vi "read log.vi"() -> ()   [LabVIEW 2020]
uses:
  <vilib>/Utility/sysdir.llb/System Directory Type.ctl
  <vilib>/addons/_JKI Toolkits/State Machine/_JKI_lib_State_Machine.llb/Select State(s)_err__jki_lib_state_machine.vi
  <vilib>/JDP Science/JSONtext/JSONtext.lvlib
panel:
  in  "refresh":bool
  in  "Log Files":i32(listbox)
  out "message":string
  in  "timestamp":i32(listbox)
  in  "Exit":bool
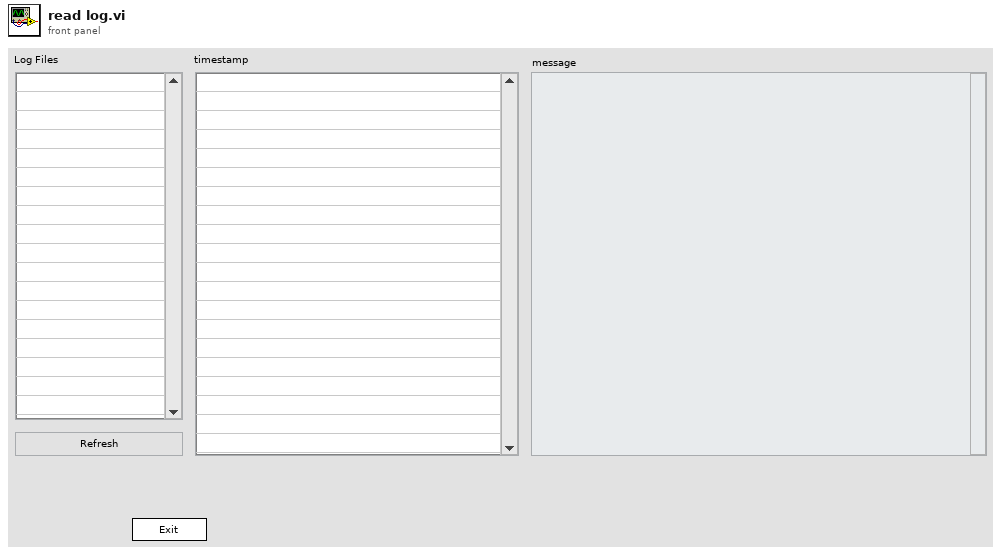
[diagram p1: front panel]
types:
  T1 = enum32{"Invalid", "Standard", "Closed", "Hidden", "Minimized", "Maximized"}
  T2 = enum32{"invalid app kind", "Development System", "Run Time System", "Student Edition", "Embedded LabVIEW", "Evaluation", "Custom"}
  T3 = cluster{"Core":cluster{"Current VI Reference":refnum<vi>, "Close Panel on Exit?":bool}, "log file":path, "elements":string[], "Log Directory":path}
  T4 = typedef "System Directory Type.ctl" = i32
  T5 = cluster{"Current VI Reference":refnum<vi>, "Close Panel on Exit?":bool}
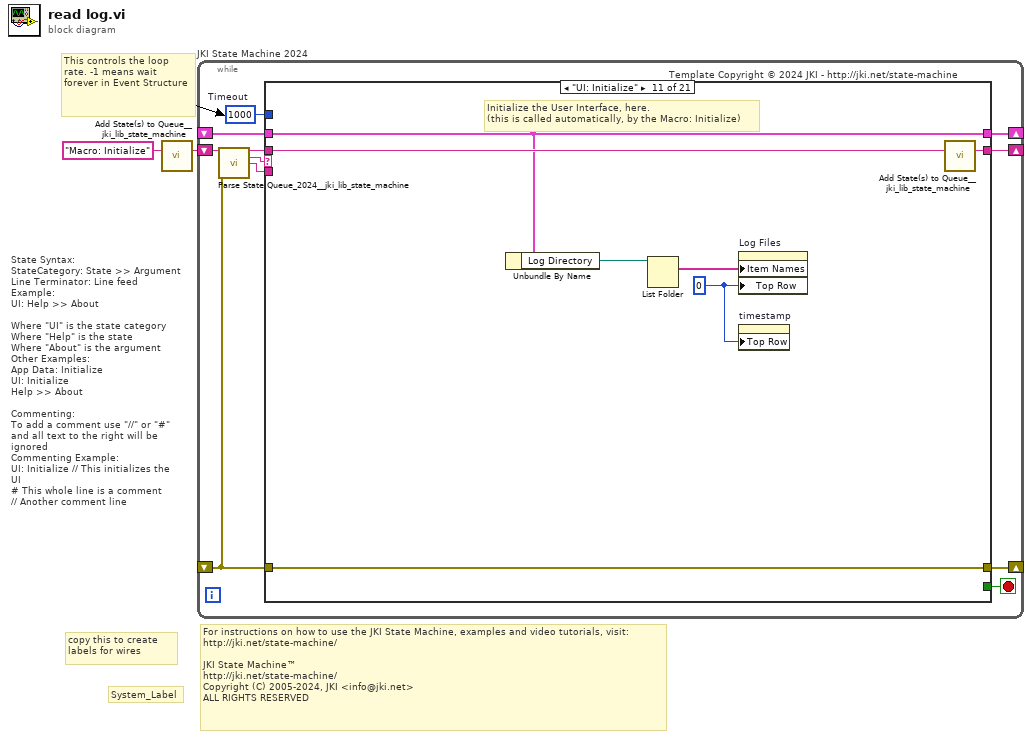
[diagram p0: block diagram]
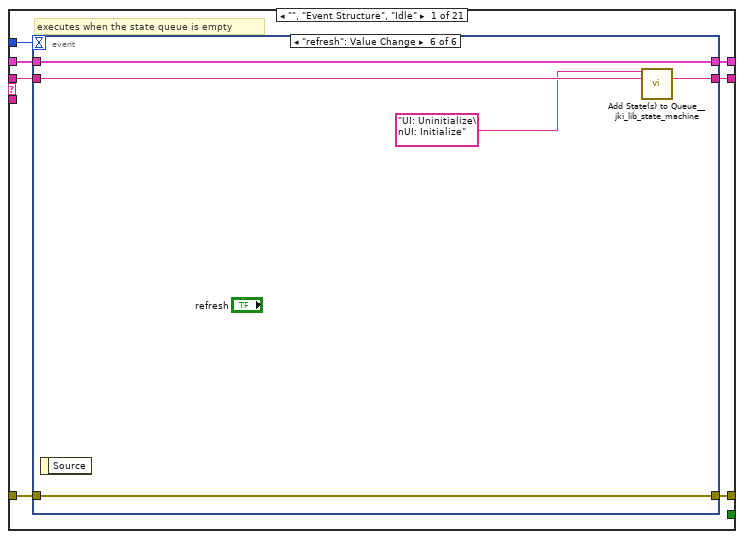
[diagram p2: hidden frame]
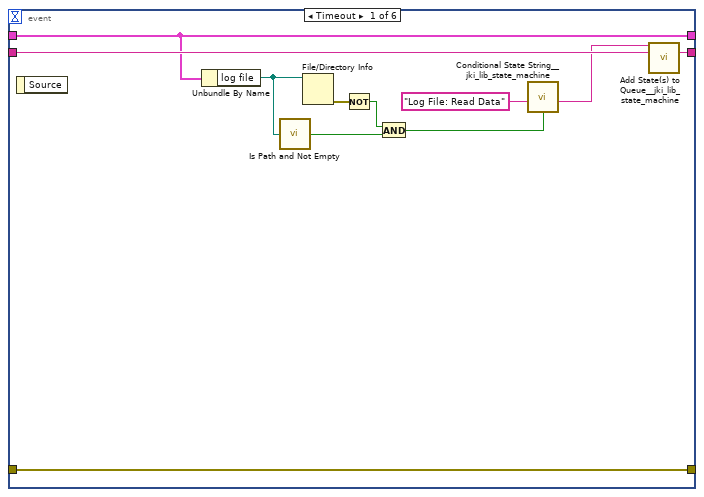
[diagram p3: hidden frame]
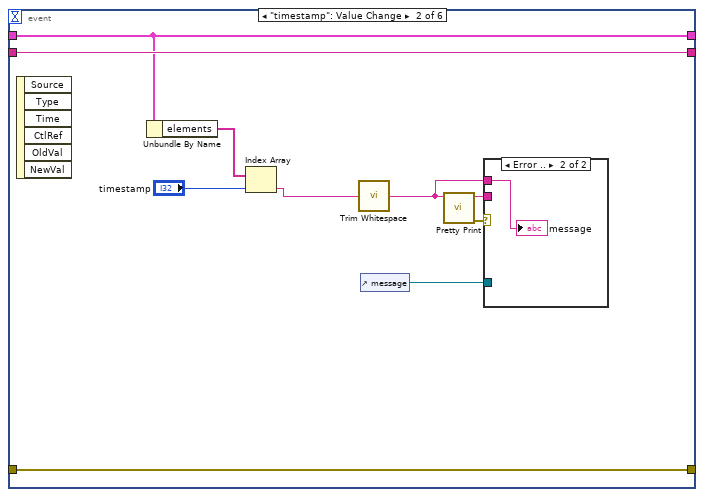
[diagram p4: hidden frame]
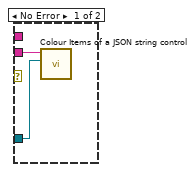
[diagram p5: hidden frame]
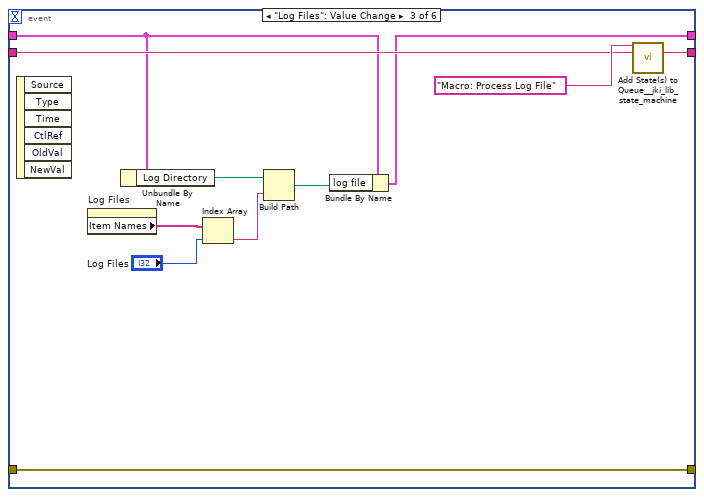
[diagram p6: hidden frame]
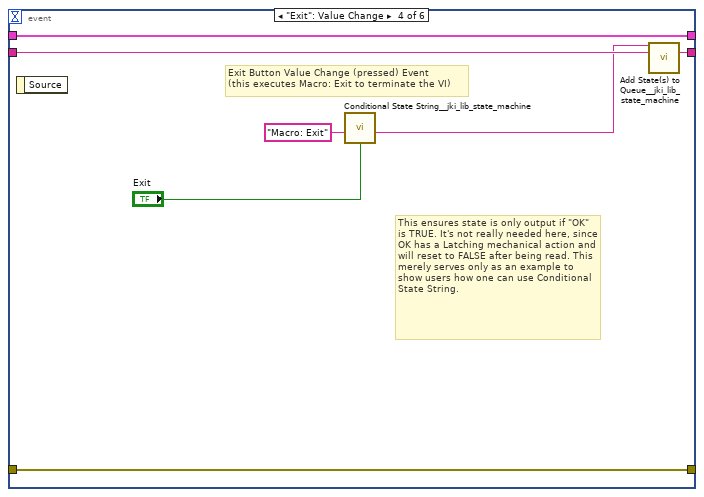
[diagram p7: hidden frame]
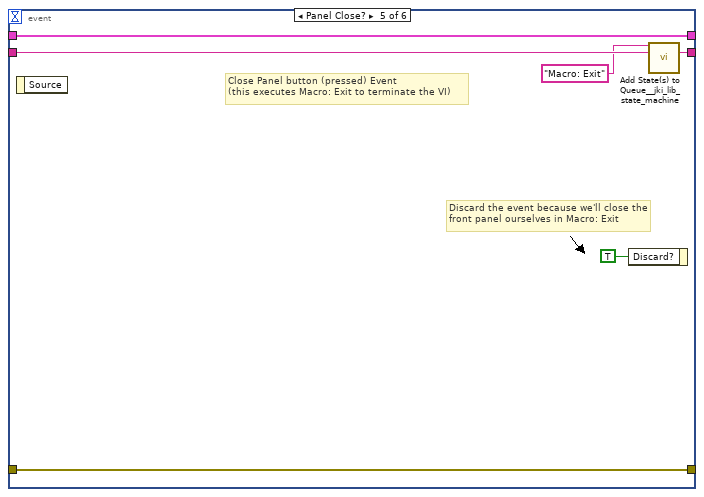
[diagram p8: hidden frame]
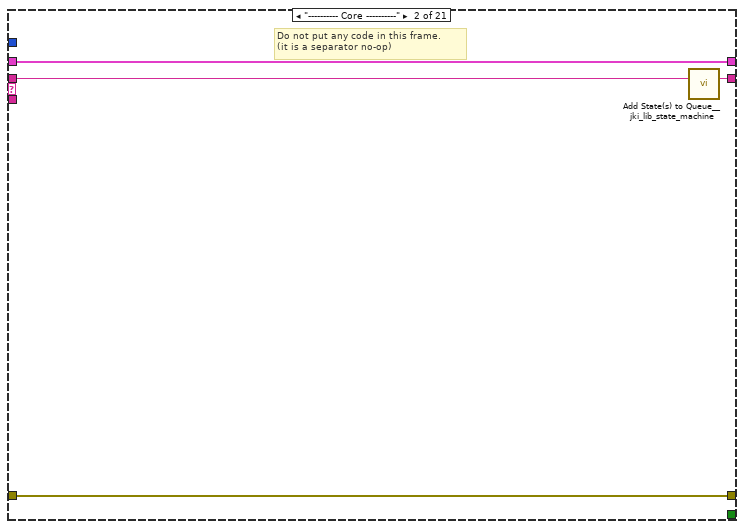
[diagram p9: hidden frame]
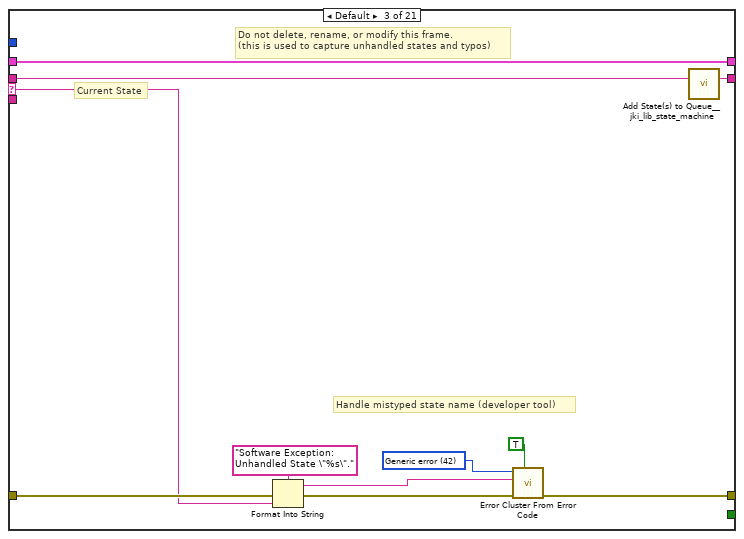
[diagram p10: hidden frame]
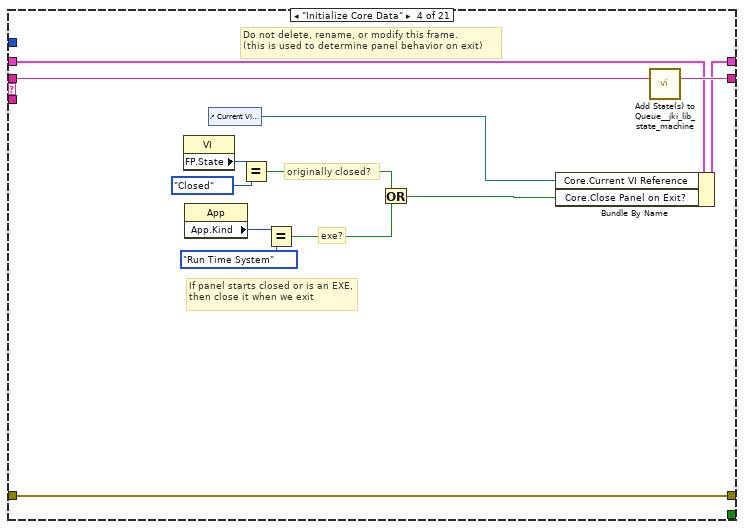
[diagram p11: hidden frame]
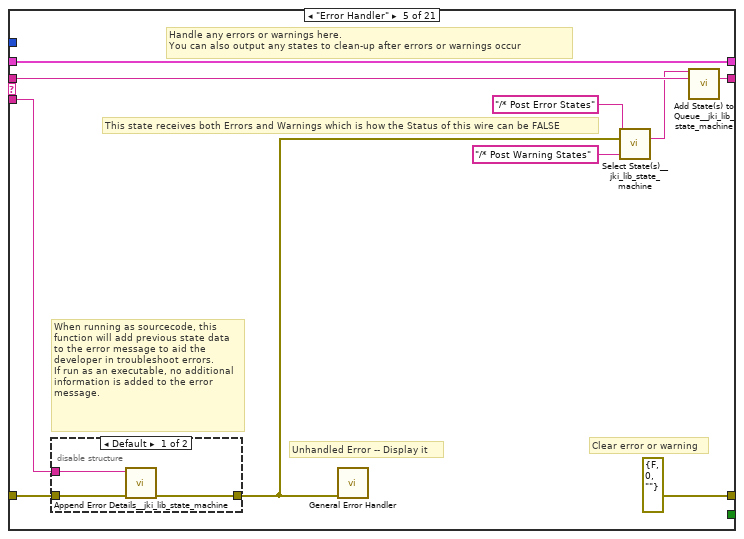
[diagram p12: hidden frame]
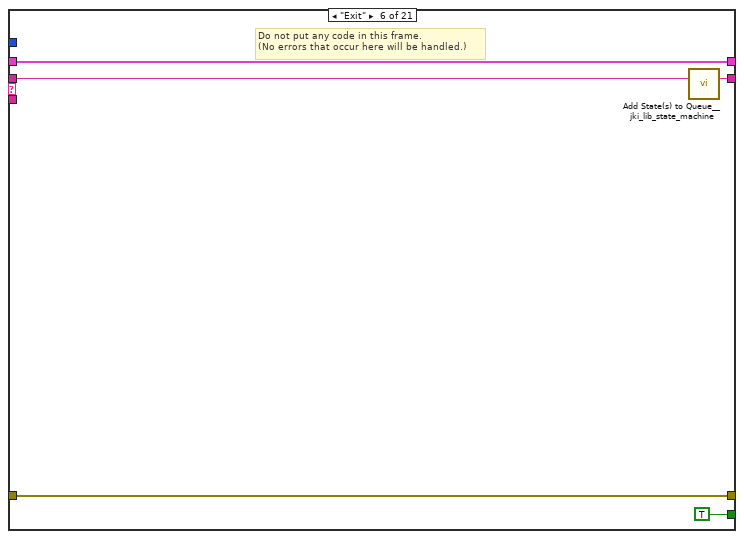
[diagram p14: hidden frame]
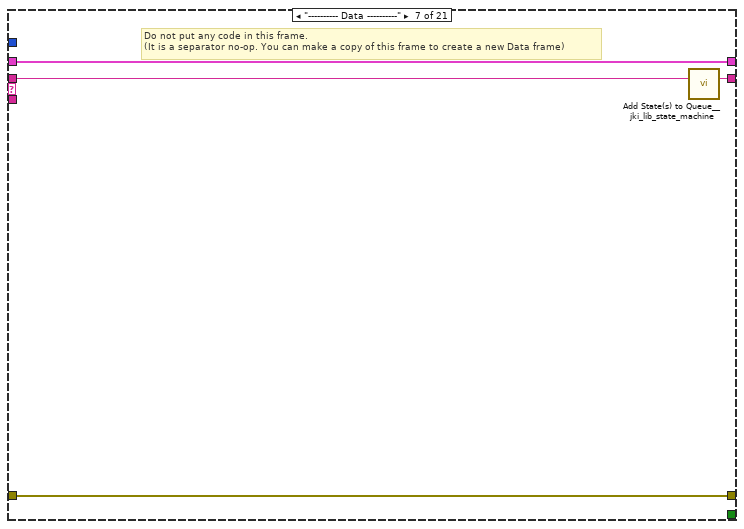
[diagram p15: hidden frame]
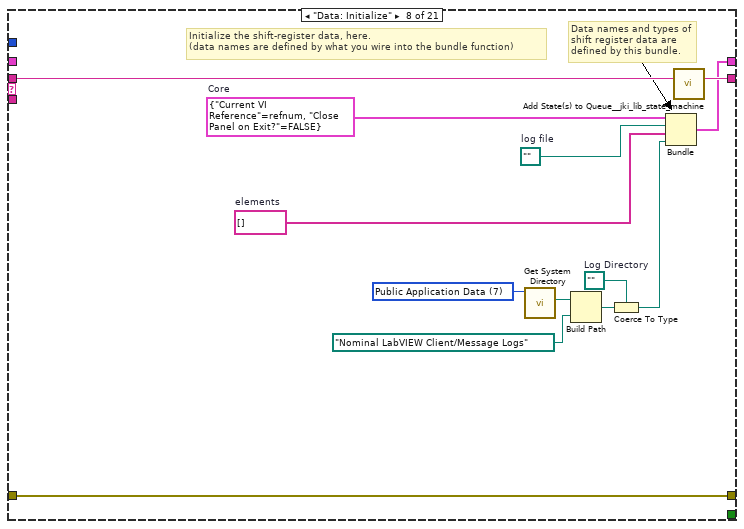
[diagram p16: hidden frame]
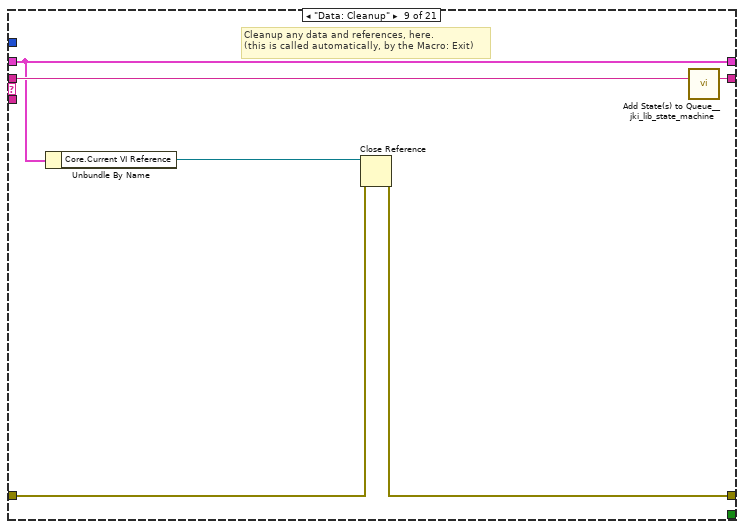
[diagram p17: hidden frame]
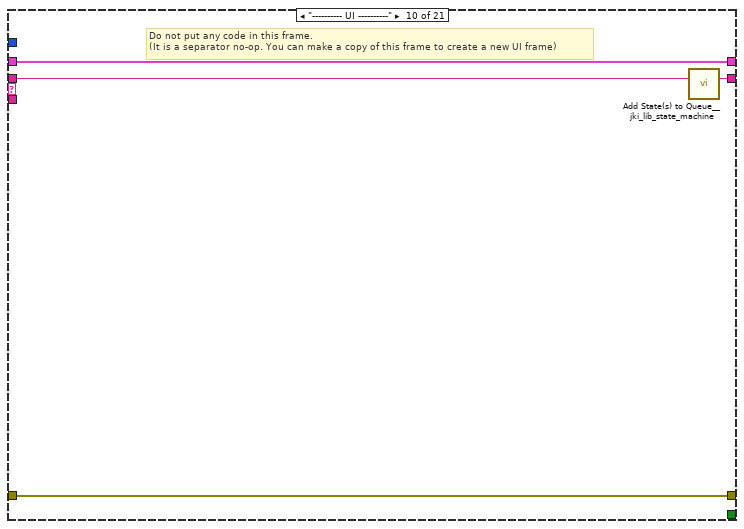
[diagram p18: hidden frame]
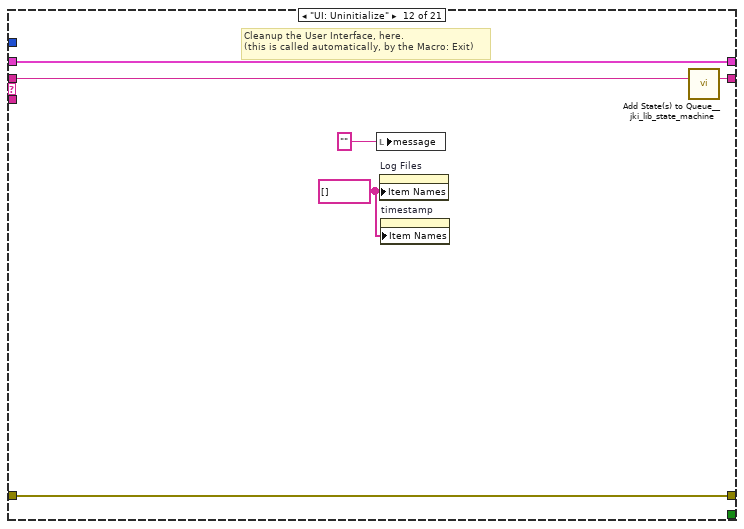
[diagram p19: hidden frame]
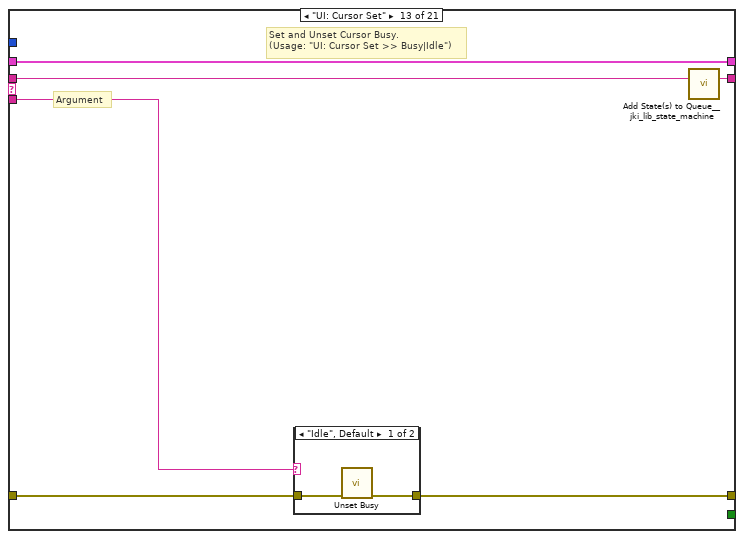
[diagram p20: hidden frame]
diagram:
  # "For instructions on how to use the JKI State Machine, examples and video tutorials, visit:\nhttp://jki.net/state-machine/\n\nJKI State Machine™\nhttp://jki.net/state-machine/\nCopyright (C) 2005-2024, JKI <info@jki.net>\nALL RIGHTS RESERVED"
  # "State Syntax:\nStateCategory: State >> Argument\nLine Terminator: Line feed\nExample:\nUI: Help >> About\n\nWhere \"UI\" is the state category\nWhere \"Help\" is the state\nWhere \"About\" is the argument\nOther Examples:\nApp Data: Initialize\nUI: Initialize\nHelp >> About\n\nCommenting:\nTo add a comment use \"//\" or \"#\" and all text to the right will be ignored\nCommenting Example:\nUI: Initialize // This initializes the UI\n# This whole line is a comment\n// Another comment line"
  # "copy this to create labels for wires"
  # "This controls the loop rate. -1 means wait forever in Event Structure"
  # "System_Label"
  n1 = call <vilib>:"Add State(s) to Queue__jki_lib_state_machine.vi"("State(s) in (\"\")"="Macro: Initialize") -> ("States Out"=w2:string)  [unwired: 14 in]
  n2 = while "JKI State Machine 2024" {
    shift-right: [w6] -> _
    shift-left: _ -> [w5]
    shift-right: [w9] -> _
    shift-left: _ -> [w3]
    shift-right: [w8] -> _
    shift-left: w2 -> [w10]
    stop <- w7 stop-if-true
    w4 = 1000  # Timeout
    # "Template Copyright © 2024 JKI - http://jki.net/state-machine"
    n3 = call <vilib>:"Parse State Queue_2024__jki_lib_state_machine.vi"("State Queue"=w10, "Error In (no error)"=w3) -> ("Remaining States"=w12:string, "Current State"=w13:string, "Arguments"=w11:string)  [unwired: 11 in]
    n4 = case shown="\"UI: Initialize\"" w13 {
      selector: w13 -> [_ _ w78 _ _ _ _ _ _ _ _ _ _ _ _ _ _ _ _ _ _]
      tunnel: w12 -> [w20 w77 w82 w101 w111 w120 w124 w137 w143 w147 w154 w155 w166 w177 w246 w251 w260 w265 w269 w285 w302]
      tunnel: w11 -> [_ _ _ _ w106 _ _ _ _ _ _ _ w161 w171 _ _ _ _ _ _ _]
      tunnel: w5 -> [w18 w74 w80 w94 w108 w118 w121 _ w138 w144 w150 w159 w164 w173 w243 w248 w258 w263 w266 w272 w299]
      tunnel: [w17 w75 w84 w98 errorcluster {"status"=FALSE, "code"=0, "source"=""} ("error out") w117 w122 w134 w139 w145 w152 w158 w162 w174 w244 w249 w255 w262 w267 w278 w300] -> w9
      tunnel: w3 -> [w14 w75 w83 w98 w107 w117 w122 w134 w140 w145 w152 w158 w163 w175 w244 w249 w255 w262 w267 w277 w300]
      tunnel: [w19 w76 w81 w100 w110 w119 w123 w136 w142 w146 w153 w160 w165 w176 w245 w250 w259 w264 w268 w284 w301] -> w8
      tunnel: [_ _ _ _ _ TRUE _ _ _ _ _ _ _ _ _ _ _ _ _ _ _] -> w7
      tunnel: [w16 w74 w80 w99 w108 w118 w121 w135 w138 w144 w150 w159 w164 w173 w243 w248 w258 w263 w266 w271 w299] -> w6
      tunnel: w4 -> [w15 _ _ _ _ _ _ _ _ _ _ _ _ _ _ _ _ _ _ _ _]
      frame "", "Event Structure", "Idle" {
        # "executes when the state queue is empty"
        n5 = event shown="[5] \"refresh\": Value Change" {
          selector: _ -> [_ _ _ _ _ _]
          dyn-events: _ -> [_ _ _ _ _ _]
          timeout: w15 -> [_ _ _ _ _ _]
          tunnel: w20 -> [w31 w41 w53 w62 w68 w71]
          tunnel: [w30 w41 w52 w61 w67 w72] -> w19
          tunnel: w18 -> [w28 w40 w47 w59 w65 w73]
          tunnel: [w29 w33 w55 w60 w66 w70] -> w17
          tunnel: w14 -> [w29 w33 w55 w60 w66 w70]
          tunnel: [w28 w40 w45 w59 w65 w73] -> w16
          event Timeout {
            n6 = event-data() -> ()  [unwired: 1 in, 1 out]
            n7 = Unbundle By Name(w28) -> ("log file"=w26:path)
            n8 = call <vilib>:"Is Path and Not Empty.vi"("path"=w26) -> ("Is Path and Not Empty?"=w25:bool)  [unwired: 4 in]
            n9 = File/Directory Info(path=w26) -> (error out=w27:errorcluster)  [unwired: 1 in, 6 out]
            n10 = Not(x=w27) -> (.not. x?=w24:bool)
            n11 = And(x=w24, y=w25) -> (x .and. y?=w22:bool)
            n12 = call <vilib>:"Conditional State String__jki_lib_state_machine.vi"("Do State(s)?"=w22, "State"="Log File: Read Data") -> ("State Out"=w23:string)  [unwired: 7 in]
            n13 = call <vilib>:"Add State(s) to Queue__jki_lib_state_machine.vi"("State(s) in Front (\"\")"=w23, "State(s) in (\"\")"=w31) -> ("States Out"=w30:string)  [unwired: 13 in]
          }
          event "timestamp": Value Change {
            n14 = event-data() -> ()  [unwired: 1 in, 6 out]
            n15 = Unbundle By Name(w40) -> ("elements"=w39:string[])
            n16 = Index Array(array=w39, index="timestamp") -> (element=w32:string)
            n17 = call <vilib>:"Trim Whitespace.vi"("string"=w32) -> ("trimmed string"=w34:string)  [unwired: 1 in]
            n18 = control-ref of="message"() -> (w37:refnum<vi>)
            n19 = call <vilib>:"Pretty Print.vi"("JSON"=w34) -> ("error out"=w35:errorcluster, "<JSON>"=w36:string)  [unwired: 8 in, 1 out]
            n20 = case shown="Error .." w35 {
              tunnel: w37 -> [w43 _]
              tunnel: w36 -> [w42 _]
              tunnel: w34 -> [_ w44]
              frame No Error {
                n21 = call <vilib>:"Colour Items of a JSON string control.vi"("String Control"=w43, "JSON"=w42) -> ()  [unwired: 9 in, 1 out]
              }
              frame Error {
                "message" <- w44
              }
            }
          }
          event "Log Files": Value Change {
            n22 = event-data() -> ()  [unwired: 1 in, 6 out]
            n23 = property on="Log Files" class="LstBox (strict)"() -> ("Item Names"=w50:string[])  [unwired: 2 in, 2 out]
            n24 = Unbundle By Name(w47) -> ("Log Directory"=w51:path)
            n25 = Index Array(array=w50, index="Log Files") -> (element=w48:string)
            n26 = Build Path(base path=w51, name or relative path=w48) -> (appended path=w46:path)
            n27 = Bundle By Name(cluster=w47, "log file"=w46) -> (w45:T3)
            n28 = call <vilib>:"Add State(s) to Queue__jki_lib_state_machine.vi"("State(s) in Front (\"\")"="Macro: Process Log File" ("string"), "State(s) in (\"\")"=w53) -> ("States Out"=w52:string)  [unwired: 13 in]
          }
          event "Exit": Value Change {
            # "This ensures state is only output if \"OK\" is TRUE. It's not really needed here, since OK has a Latching mechanical action and will reset to FALSE after being read. This merely serves only as an example to show users how one can use Conditional State String."
            # "Exit Button Value Change (pressed) Event\n(this executes Macro: Exit to terminate the VI)"
            n29 = event-data() -> ()  [unwired: 1 in, 1 out]
            n30 = call <vilib>:"Conditional State String__jki_lib_state_machine.vi"("Do State(s)?"="Exit", "State"="Macro: Exit") -> ("State Out"=w56:string)  [unwired: 7 in]
            n31 = call <vilib>:"Add State(s) to Queue__jki_lib_state_machine.vi"("State(s) in Front (\"\")"=w56, "State(s) in (\"\")"=w62) -> ("States Out"=w61:string)  [unwired: 13 in]
          }
          event Panel Close? {
            # "Discard the event because we'll close the front panel ourselves in Macro: Exit"
            # "Close Panel button (pressed) Event\n(this executes Macro: Exit to terminate the VI)"
            n32 = event-data() -> ()  [unwired: 1 in, 1 out]
            n33 = event-data("Discard?"=TRUE) -> ()  [unwired: 1 in, 1 out]
            n34 = call <vilib>:"Add State(s) to Queue__jki_lib_state_machine.vi"("State(s) in Front (\"\")"="Macro: Exit", "State(s) in (\"\")"=w68) -> ("States Out"=w67:string)  [unwired: 13 in]
          }
          event "refresh": Value Change {
            n35 = event-data() -> ()  [unwired: 1 in, 1 out]
            n36 = call <vilib>:"Add State(s) to Queue__jki_lib_state_machine.vi"("State(s) in Front (\"\")"="UI: Uninitialize\nUI: Initialize" ("State(s) in Front (\"\")"), "State(s) in (\"\")"=w71) -> ("States Out"=w72:string)  [unwired: 13 in]
          }
        }
      }
      frame "---------- Core ----------" {
        # "Do not put any code in this frame.\n(it is a separator no-op)"
        n37 = call <vilib>:"Add State(s) to Queue__jki_lib_state_machine.vi"("State(s) in (\"\")"=w77) -> ("States Out"=w76:string)  [unwired: 14 in]
      }
      frame Default {
        w87 = 42 items=["No error", "Argument error", "Memory is full", "Out of zone", "End of file", "File already open", "Generic file I/O error", "File not found", "File permission error", "Disk is full", "Duplicate path", "Too many files open", "System feature not enabled", "Resource file not found", "Cannot add resource", "Resource not found", "Image not found", "Image memory error", "Pen does not exist", "Config type invalid", "Config token not found", "Config parse error", "Config memory error", "Bad external code format", "Bad external code offset", "External code not present", "Null window", "Destroy window error", "Null menu", "Print aborted", "Bad print record", "Print driver error", "Windows error during printing", "Memory error during printing", "Print dialog error", "Generic print error", "Invalid device refnum", "Device not found", "Device parameter error", "Device unit error", "Cannot open device", "Device call aborted", "Generic error", "Cancelled by user", "Object ID too low", "Object ID too high", "Object not in heap", "Unknown heap", "Unknown object (invalid DefProc)", "Unknown object (DefProc not in table)", "Message out of range", "Invalid (null) method", "Unknown message", "Manager call not supported", "Bad address", "Network operation in progress", "Network operation timed out", "Connection is busy", "Network attribute not supported", "Network error", "Address in use", "System out of memory", "Connection aborted", "Connection refused", "Not connected", "Already connected", "Connection closed", "Initialization error (interapplication manager)", "Bad occurrence", "Wait on unbound occurrence handler", "Occurrence queue overflow", "Datalog type conflict", "Unused", "Unrecognized type (interapplication manager)", "Memory corrupt", "Failed to make temporary DLL", "Old CIN version", "Drag socket not found", "Failed to load drop-object", "Failed to register OLE object", "Failed to release OLE object", "Format specifier type mismatch", "Unknown format specifier", "Too few format specifiers", "Too many format specifiers", "Scan failed", "Newer CIN version", "Error converting to variant", "Runtime menu error", "Password tampered", "Variant attribute not found", "Incompatible variant data type", "Event data is not available", "Event Store is not present", "Occurrence is not found", "Event Queue is not created", "Event info is not available", "Refnum passed is NULL", "Error retrieving Class GUID", "Error retrieving CoClass GUID", "Error retrieving TypeLib GUID.", "Bad built application magic bytes.", "Specific driver is different from the specific driver associated with the Logical Name.", "There is no session opened to the class driver.", "Max Error", "MAX - Error with config objects", "MAX - Error loading configuration", "MAX - Group not supported"]
        # "Current State"
        # "Do not delete, rename, or modify this frame.\n(this is used to capture unhandled states and typos)"
        # "Handle mistyped state name (developer tool)"
        n38 = Format Into String(format string="Software Exception: Unhandled State \"%s\"." ("message"), error in=w83, w78) -> (resulting string=w86:string, error out=w85:errorcluster)  [unwired: 1 in]
        n39 = call <vilib>:"Error Cluster From Error Code.vi"("show call chain? (False)"=TRUE, "error in (no error)"=w85, "error message (\"\")"=w86, "error code (0)"=w87) -> ("error out"=w84:errorcluster)  [unwired: 5 in]
        n40 = call <vilib>:"Add State(s) to Queue__jki_lib_state_machine.vi"("State(s) in (\"\")"=w82) -> ("States Out"=w81:string)  [unwired: 14 in]
      }
      frame "Initialize Core Data" {
        # "Do not delete, rename, or modify this frame.\n(this is used to determine panel behavior on exit)"
        # "originally closed?"
        # "exe?"
        # "If panel starts closed or is an EXE, then close it when we exit"
        n41 = property class="VI"() -> ("FP.State"=w91:T1)  [unwired: 2 in, 2 out]
        n42 = property class="App"() -> ("App.Kind"=w97:T2)  [unwired: 2 in, 2 out]
        n43 = control-ref of="Current VI Reference"() -> (w92:refnum<vi>)
        n44 = Equal?(x=w91, y=T1."Closed" ("Front Panel Window:State")) -> (x = y?=w89:bool)
        n45 = Equal?(x=w97, y=T2."Run Time System" ("Application:Kind")) -> (x = y?=w95:bool)
        n46 = Or(x=w89, y=w95) -> (x .or. y?=w93:bool)
        n47 = Bundle By Name(cluster=w94, "Core.Current VI Reference"=w92, "Core.Close Panel on Exit?"=w93) -> (w99:T3)
        n48 = call <vilib>:"Add State(s) to Queue__jki_lib_state_machine.vi"("State(s) in (\"\")"=w101) -> ("States Out"=w100:string)  [unwired: 14 in]
      }
      frame "Error Handler" {
        # "When running as sourcecode, this function will add previous state data to the error message to aid the developer in troubleshoot errors.\nIf run as an executable, no additional information is added to the error message."
        # "This state receives both Errors and Warnings which is how the Status of this wire can be FALSE"
        # "Unhandled Error -- Display it"
        # "Handle any errors or warnings here.\nYou can also output any states to clean-up after errors or warnings occur"
        # "Clear error or warning"
        n49 = disable-structure shown="Default" {
          disable-tunnel: w107 -> [w114 w115]
          disable-tunnel: w106 -> [w113 _]
          disable-tunnel: [w112 w115] -> w105
          frame condition #0 (active) {
            n50 = call <vilib>:"Append Error Details__jki_lib_state_machine.vi"("error in (no error)"=w114, "Previous State and Argument(s)"=w113) -> ("error out"=w112:errorcluster)  [unwired: 9 in]
          }
          frame condition #1 {
          }
        }
        n51 = call <vilib>:"General Error Handler.vi"("error in (no error)"=w105) -> ()  [unwired: 10 in, 5 out]
        n52 = call-poly <vilib>:"Select State(s)__jki_lib_state_machine.vi"("State(s) if True (\"\")"="/* Post Error States", "Select"=w105, "State(s) if False (\"\")"="/* Post Warning States") -> ("States Out"=w103:string)  [unwired: 12 in]
        n53 = call <vilib>:"Add State(s) to Queue__jki_lib_state_machine.vi"("State(s) in Front (\"\")"=w103, "State(s) in (\"\")"=w111) -> ("States Out"=w110:string)  [unwired: 13 in]
      }
      frame "Exit" {
        # "Do not put any code in this frame.\n(No errors that occur here will be handled.)"
        n54 = call <vilib>:"Add State(s) to Queue__jki_lib_state_machine.vi"("State(s) in (\"\")"=w120) -> ("States Out"=w119:string)  [unwired: 14 in]
      }
      frame "---------- Data ----------" {
        # "Do not put any code in this frame.\n(It is a separator no-op. You can make a copy of this frame to create a new Data frame)"
        n55 = call <vilib>:"Add State(s) to Queue__jki_lib_state_machine.vi"("State(s) in (\"\")"=w124) -> ("States Out"=w123:string)  [unwired: 14 in]
      }
      frame "Data: Initialize" {
        w125 = path ""  # Log Directory
        w130 = T4 7 items=["User Home"=0, "User Desktop"=1, "User Documents"=2, "User Application Data"=3, "User Preferences"=4, "User Temporary"=5, "Public Documents"=6, "Public Application Data"=7, "Public Preferences"=8, "Public Cache"=13, "System Core Libraries"=9, "System Installed Libraries"=10, "Application Files"=11, "Boot Volume Root"=12] ("system directory type")
        w131 = string[] []  # elements
        w132 = path ""  # log file
        w133 = T5 {"Current VI Reference"=refnum, "Close Panel on Exit?"=FALSE}  # Core
        # "Data names and types of shift register data are defined by this bundle."
        # "Initialize the shift-register data, here.\n(data names are defined by what you wire into the bundle function)"
        n56 = call <vilib>:"Get System Directory.vi"("system directory type"=w130) -> ("system directory"=w129:path)  [unwired: 10 in]
        n57 = Build Path(base path=w129, name or relative path=path "Nominal LabVIEW Client/Message Logs") -> (appended path=w127:path)
        n58 = Coerce To Type(0:w127, 1:w125) -> (2:w126:path)
        n59 = Bundle("Core"=w133, "log file"=w132, "elements"=w131, "Log Directory"=w126) -> (w135:T3)  [unwired: 1 in]
        n60 = call <vilib>:"Add State(s) to Queue__jki_lib_state_machine.vi"("State(s) in (\"\")"=w137) -> ("States Out"=w136:string)  [unwired: 14 in]
      }
      frame "Data: Cleanup" {
        # "Cleanup any data and references, here.\n(this is called automatically, by the Macro: Exit)"
        n61 = Unbundle By Name(w138) -> ("Core.Current VI Reference"=w141:refnum<vi>)
        n62 = Close Reference(reference=w141, error in (no error)=w140) -> (error out=w139:errorcluster)
        n63 = call <vilib>:"Add State(s) to Queue__jki_lib_state_machine.vi"("State(s) in (\"\")"=w143) -> ("States Out"=w142:string)  [unwired: 14 in]
      }
      frame "---------- UI ----------" {
        # "Do not put any code in this frame.\n(It is a separator no-op. You can make a copy of this frame to create a new UI frame)"
        n64 = call <vilib>:"Add State(s) to Queue__jki_lib_state_machine.vi"("State(s) in (\"\")"=w147) -> ("States Out"=w146:string)  [unwired: 14 in]
      }
      frame "UI: Initialize" {
        w148 = 0 ("Top Row")
        # "Initialize the User Interface, here.\n(this is called automatically, by the Macro: Initialize)"
        n65 = Unbundle By Name(w150) -> ("Log Directory"=w149:path)
        n66 = List Folder(path=w149) -> (filenames=w151:string[])  [unwired: 3 in, 3 out]
        n67 = property on="Log Files" class="LstBox (strict)"("Item Names"=w151, "Top Row"=w148) -> ()  [unwired: 2 in, 2 out]
        n68 = property on="timestamp" class="LstBox (strict)"("Top Row"=w148) -> ()  [unwired: 2 in, 2 out]
        n69 = call <vilib>:"Add State(s) to Queue__jki_lib_state_machine.vi"("State(s) in (\"\")"=w154) -> ("States Out"=w153:string)  [unwired: 14 in]
      }
      frame "UI: Uninitialize" {
        w157 = string[] [] ("Item Names")
        # "Cleanup the User Interface, here.\n(this is called automatically, by the Macro: Exit)"
        n70 = local write "message"("") -> ()
        n71 = property on="Log Files" class="LstBox (strict)"("Item Names"=w157) -> ()  [unwired: 2 in, 2 out]
        n72 = property on="timestamp" class="LstBox (strict)"("Item Names"=w157) -> ()  [unwired: 2 in, 2 out]
        n73 = call <vilib>:"Add State(s) to Queue__jki_lib_state_machine.vi"("State(s) in (\"\")"=w155) -> ("States Out"=w160:string)  [unwired: 14 in]
      }
      frame "UI: Cursor Set" {
        # "Argument"
        # "Set and Unset Cursor Busy.\n(Usage: \"UI: Cursor Set >> Busy|Idle\")"
        n74 = case shown="\"Idle\", Default" w161 {
          tunnel: w163 -> [w168 w170]
          tunnel: [w167 w169] -> w162
          frame "Idle", Default {
            n75 = call <vilib>:"Unset Busy.vi"("error in (no error)"=w168) -> ("error out"=w167:errorcluster)  [unwired: 10 in]
          }
          frame "Busy" {
            n76 = call <vilib>:"Set Busy.vi"("error in (no error)"=w170) -> ("error out"=w169:errorcluster)  [unwired: 9 in, 1 out]
          }
        }
        n77 = call <vilib>:"Add State(s) to Queue__jki_lib_state_machine.vi"("State(s) in (\"\")"=w166) -> ("States Out"=w165:string)  [unwired: 14 in]
      }
      frame "UI: Front Panel State" {
        # "Argument"
        # "Set Front Panel Open or Closed\n(Usage: \"UI: Front Panel State >> Open|Close\")"
        n78 = Unbundle By Name(w173) -> ("Core.Current VI Reference"=w172:refnum<vi>)
        n79 = case shown="\"Minimize\", \"Minimized\"" w171 {
          tunnel: w175 -> [w183 w198 w209 w222 w235]
          tunnel: [w185 w199 w211 w224 w237] -> w174
          tunnel: w172 -> [w184 w196 w210 w223 w236]
          frame "Open", "Standard", Default {
            w178 = T1."Standard" ("State")
            n80 = property class="VI"(reference=w184, error in=w183) -> (reference out=w181:refnum<vi>, error out=w182:errorcluster, "FP.State"=w180:T1)
            n81 = Not Equal?(x=w180, y=w178) -> (x != y?=w179:bool)
            n82 = case shown="True" w179 {
              tunnel: [w189 w191] -> w185
              tunnel: w182 -> [w188 w191]
              tunnel: w181 -> [w187 _]
              tunnel: w178 -> [w186 _]
              frame True {
                n83 = invoke class="VI" method="FP.Open"(reference=w187, error in=w188, "Activate"=TRUE, "State"=w186) -> (error out=w189:errorcluster)  [unwired: 1 in, 4 out]
              }
              frame False {
              }
            }
          }
          frame "Close", "Closed" {
            n84 = property class="VI"(reference=w196, error in=w198) -> (reference out=w195:refnum<vi>, error out=w197:errorcluster, "FP.State"=w193:T1)
            n85 = Not Equal?(x=w193, y=T1."Closed" ("Front Panel Window:State")) -> (x != y?=w192:bool)
            n86 = case shown="True" w192 {
              tunnel: [w200 w203] -> w199
              tunnel: w197 -> [w200 w202]
              tunnel: w195 -> [_ w201]
              frame False {
              }
              frame True {
                n87 = invoke class="VI" method="FP.Close"(reference=w201, error in=w202) -> (error out=w203:errorcluster)  [unwired: 1 in, 2 out]
              }
            }
          }
          frame "Hidden", "Hide" {
            w204 = T1."Hidden" ("State")
            n88 = property class="VI"(reference=w210, error in=w209) -> (reference out=w207:refnum<vi>, error out=w208:errorcluster, "FP.State"=w206:T1)
            n89 = Not Equal?(x=w206, y=w204) -> (x != y?=w205:bool)
            n90 = case shown="True" w205 {
              tunnel: [w215 w216] -> w211
              tunnel: w208 -> [w214 w216]
              tunnel: w207 -> [w213 _]
              tunnel: w204 -> [w212 _]
              frame True {
                n91 = invoke class="VI" method="FP.Open"(reference=w213, error in=w214, "State"=w212) -> (error out=w215:errorcluster)  [unwired: 2 in, 4 out]
              }
              frame False {
              }
            }
          }
          frame "Minimize", "Minimized" {
            w217 = T1."Minimized" ("State")
            n92 = property class="VI"(reference=w223, error in=w222) -> (reference out=w220:refnum<vi>, error out=w221:errorcluster, "FP.State"=w219:T1)
            n93 = Not Equal?(x=w219, y=w217) -> (x != y?=w218:bool)
            n94 = case shown="True" w218 {
              tunnel: [w228 w229] -> w224
              tunnel: w221 -> [w227 w229]
              tunnel: w220 -> [w226 _]
              tunnel: w217 -> [w225 _]
              frame True {
                n95 = invoke class="VI" method="FP.Open"(reference=w226, error in=w227, "State"=w225) -> (error out=w228:errorcluster)  [unwired: 2 in, 4 out]
              }
              frame False {
              }
            }
          }
          frame "Maximize", "Maximized" {
            w230 = T1."Maximized" ("State")
            n96 = property class="VI"(reference=w236, error in=w235) -> (reference out=w233:refnum<vi>, error out=w234:errorcluster, "FP.State"=w232:T1)
            n97 = Not Equal?(x=w232, y=w230) -> (x != y?=w231:bool)
            n98 = case shown="True" w231 {
              tunnel: [w241 w242] -> w237
              tunnel: w234 -> [w240 w242]
              tunnel: w233 -> [w239 _]
              tunnel: w230 -> [w238 _]
              frame True {
                n99 = invoke class="VI" method="FP.Open"(reference=w239, error in=w240, "State"=w238) -> (error out=w241:errorcluster)  [unwired: 2 in, 4 out]
              }
              frame False {
              }
            }
          }
        }
        n100 = call <vilib>:"Add State(s) to Queue__jki_lib_state_machine.vi"("State(s) in (\"\")"=w177) -> ("States Out"=w176:string)  [unwired: 14 in]
      }
      frame "---------- Macro ----------" {
        # "Do not put any code in this frame.\n(It is a separator no-op. You can make a copy of this frame to create a new Macro frame)"
        n101 = call <vilib>:"Add State(s) to Queue__jki_lib_state_machine.vi"("State(s) in (\"\")"=w246) -> ("States Out"=w245:string)  [unwired: 14 in]
      }
      frame "Macro: Initialize" {
        w247 = "Data: Initialize\nInitialize Core Data\nUI: Initialize\nUI: Front Panel State >> Open"  # Data: Initialize Initialize Core Data UI: Initialize UI: Front Panel State >> Open
        # "Initialization Macro\n(This is called once, when the VI starts)"
        n102 = call <vilib>:"Add State(s) to Queue__jki_lib_state_machine.vi"("State(s) in Front (\"\")"=w247, "State(s) in (\"\")"=w251) -> ("States Out"=w250:string)  [unwired: 13 in]
      }
      frame "Macro: Exit" {
        # "Exit Macro\n(This is called once, when the VI exits)"
        n103 = Unbundle By Name(w258) -> ("Core.Close Panel on Exit?"=w253:bool)
        n104 = call <vilib>:"Conditional State String__jki_lib_state_machine.vi"("Do State(s)?"=w253, "State"="UI: Front Panel State >> Close") -> ("State Out"=w252:string)  [unwired: 7 in]
        n105 = call <vilib>:"Add State(s) to Queue__jki_lib_state_machine.vi"("State(s) in (\"\")"=w252, "State(s) at Back (\"\")"="UI: Uninitialize\nData: Cleanup\nExit") -> ("States Out"=w256:string)  [unwired: 13 in]
        n106 = call <vilib>:"Add State(s) to Queue__jki_lib_state_machine.vi"("State(s) in Front (\"\")"=w256, "State(s) in (\"\")"=w260) -> ("States Out"=w259:string)  [unwired: 13 in]
      }
      frame "Macro: Process Log File" {
        # "Exit Macro\n(This is called once, when the VI exits)"
        n107 = call <vilib>:"Add State(s) to Queue__jki_lib_state_machine.vi"("State(s) in Front (\"\")"="Log File: Read Data" ("State(s) in Front (\"\")"), "State(s) in (\"\")"=w265) -> ("States Out"=w264:string)  [unwired: 13 in]
      }
      frame "---------- Log File ----------" {
        # "Template Separator\n(You can make a copy of, or modify, this frame)"
        n108 = call <vilib>:"Add State(s) to Queue__jki_lib_state_machine.vi"("State(s) in (\"\")"=w269) -> ("States Out"=w268:string)  [unwired: 14 in]
      }
      frame "Log File: Read Data" {
        # "Your code here.\n(You can make a copy of, or modify, this frame)"
        n109 = Unbundle By Name(w272) -> ("log file"=w283:path)
        n110 = Open/Create/Replace File(file path (use dialog)=w283, error in=w277) -> (refnum out=w282:refnum<file>, error out=w280:errorcluster)  [unwired: 4 in, 1 out]
        n111 = Read from Text File(file (use dialog)=w282, error in=w280) -> (refnum out=w281:refnum<file>, text=w275:string, error out=w279:errorcluster)  [unwired: 2 in, 1 out]
        n112 = Close File(refnum=w281, error in=w279) -> (error out=w278:errorcluster)  [unwired: 1 out]
        n113 = call <vilib>:"Delimited String to 1D String Array.vi"("delimiter"="\n\n=*=*=*=*=*=*=*=*=*=*=*=*=*=*=*=*=*=*=*=*=*=*=*=*=*=*=*=\n", "delimited string"=w275) -> ("string array"=w274:string[])  [unwired: 9 in]
        n114 = for {
          tunnel: w274 -> [w294] mode=indexing
          tunnel: [w286] -> w270 mode=indexing if=w291
          tunnel: [w287] -> w273 mode=indexing if=w291
          (unwired) "%<%Y-%m-%d_%.3X>T" ("format string")
          n115 = call <vilib>:"Trim Whitespace.vi"("string"=w294) -> ("trimmed string"=w293:string)  [unwired: 1 in]
          n116 = Empty String/Path?(string/path=w293) -> (empty?=w292:bool)
          n117 = call <vilib>:"Delimited String to 1D String Array.vi"("delimiter"="\n", "delimited string"=w293) -> ("string array"=w297:string[])  [unwired: 9 in]
          n118 = Not(x=w292) -> (.not. x?=w291:bool)
          n119 = Delete From Array(array=w297) -> (deleted portion=w296:string)  [unwired: 2 in, 1 out]
          n120 = Index Array(array=w297) -> (element #1=w289:string, element #2=w288:string)  [unwired: 2 in]
          n121 = Match Pattern(string=w296, regular expression=": " ("search string/char (-)")) -> (after substring=w286:string)  [unwired: 1 in, 3 out]
          n122 = Format Into String(format string="%s: %s", w289, w288) -> (resulting string=w287:string)  [unwired: 2 in, 1 out]
        }
        n123 = property on="timestamp" class="LstBox (strict)"("Item Names"=w273) -> ()  [unwired: 2 in, 2 out]
        n124 = Bundle By Name(cluster=w272, "elements"=w270) -> (w271:T3)
        n125 = call <vilib>:"Add State(s) to Queue__jki_lib_state_machine.vi"("State(s) in (\"\")"=w285) -> ("States Out"=w284:string)  [unwired: 14 in]
      }
      frame "New Category: 2" {
        # "Your code here.\n(You can make a copy of, or modify, this frame)"
        n126 = call <vilib>:"Add State(s) to Queue__jki_lib_state_machine.vi"("State(s) in (\"\")"=w302) -> ("States Out"=w301:string)  [unwired: 14 in]
      }
    }
  }
